vi "TriggerTests_1_2.vi"() -> ()   [LabVIEW 2009]
uses:
  <vilib>/Utility/NIReport.llb/NI_report.lvclass
  <vilib>/express/express signal manip/GetorSetDDTAttributes/Set DDT Attributes/Set DDT Properties.xnode
  <vilib>/express/express shared/transition.llb/Waveform Array To Dynamic.vi
  <vilib>/express/express signal manip/GetorSetDDTAttributes/Set DDT Attributes/SetT0.vi
  <vilib>/express/express shared/transition.llb/Dynamic To Waveform Array.vi
  <vilib>/express/express signal manip/GetorSetDDTAttributes/Shared VIs/XDimension Enum to String.vi
  <vilib>/express/express signal manip/GetorSetDDTAttributes/Shared VIs/XDimension.ctl
  <vilib>/express/express signal manip/GetorSetDDTAttributes/Shared VIs/GetSetShared.lvlib
panel:
  in  "Report Enable":bool=TRUE
  in  "Curve data path":path=path "D:/CTA/IntegrationBoard/tmp"
  in  "Instrument VISA in":T1={"AWG VISA"="81160A", "Oscilloscope  VISA "="DSO80204B", "Integration Board IP"="172.16.7.43", "connection ID"=refnum, "report out"=refnum}
  out "error out":errorcluster
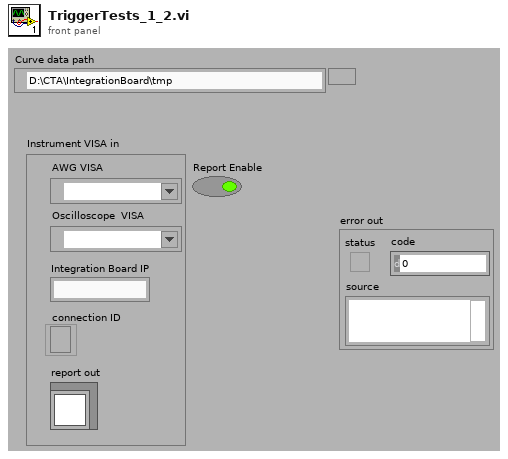
[diagram p1: front panel]
types:
  T1 = cluster{"AWG VISA":refnum<visa-resource-name>, "Oscilloscope  VISA ":refnum<visa-resource-name>, "Integration Board IP":string, "connection ID":refnum<k5>, "report out":refnum<class "NI_report.lvclass">}
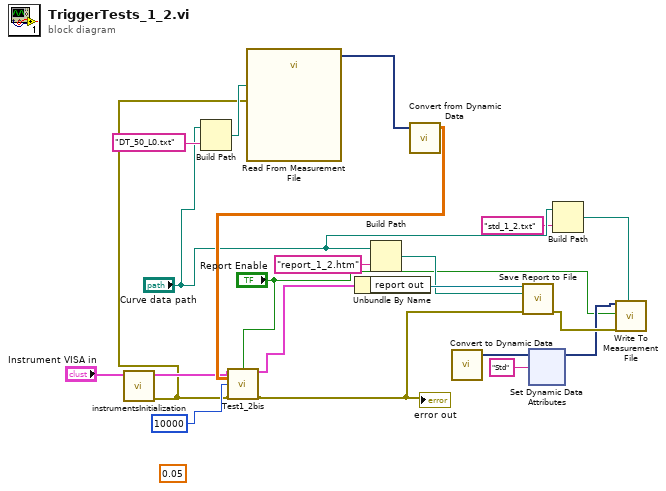
[diagram p0: block diagram]
diagram:
  (unwired) 0.05 ("Voltage Step")
  n1 = call "instrumentsInitialization.vi"("Instrument VISA in"="Instrument VISA in") -> ("error out"=w5:errorcluster, "Instrument VISA out"=w7:T1)  [unwired: 9 in]
  n2 = Build Path(base path="Curve data path", name or relative path="DT_50_L0.txt" ("Comment")) -> (appended path=w12:path)
  n3 = call "Read From Measurement File"("error in (no error)"=w5, "Filename"=w12) -> ("Signals"=w11:dynamicdata)  [unwired: 4 in, 5 out]
  n4 = Build Path(base path="Curve data path", name or relative path="report_1_2.htm") -> (appended path=w17:path)
  n5 = call "Convert from Dynamic Data"("Dynamic Data Type"=w11) -> ("Array"=w10:dbl[][])  [unwired: 3 in]
  n6 = call "Test1_2bis.vi"("Instrument VISA in"=w7, "Report Enable"="Report Enable", "DT_50_L0"=w10, "Cycles Burst"=10000, "error in"=w5) -> ("Instrument VISA out"=w8:T1, "error out"=w4:errorcluster)  [unwired: 9 in]
  "error out" <- w4
  n7 = Unbundle By Name(w8) -> ("report out"=w20:refnum<class "NI_report.lvclass">)
  n8 = call "Convert to Dynamic Data"() -> ("Dynamic Data Type"=w15:dynamicdata)  [unwired: 4 in]
  n9 = call-dynamic "Save Report to File.vi"("report in"=w20, "report file path"=w17, "error in (no error)"=w4) -> ("error out"=w19:errorcluster)  [unwired: 11 in, 1 out]
  n10 = xnode ("Set Dynamic Data Attributes")("Signals In"=w15, "Signal Name"="Std") -> ("Signals Out"=w14:dynamicdata)  [unwired: 3 in, 1 out]
  n11 = Build Path(base path="Curve data path", name or relative path="std_1_2.txt") -> (appended path=w1:path)
  n12 = call "Write To Measurement File"("Signals"=w14, "Enable"="Report Enable", "error in (no error)"=w19, "Filename"=w1) -> ()  [unwired: 13 in, 3 out]
